vi "get_and_insert_SN.vi"(8 "error in (no error)":errorcluster, 10 "read buffer in":string, 11 "VISA Refnum in":refnum<visa-resource-name>) -> (0 "error out":errorcluster, 2 "read buffer out":string, 3 "VISA Refnum out":refnum<visa-resource-name>)   [LabVIEW 2015]
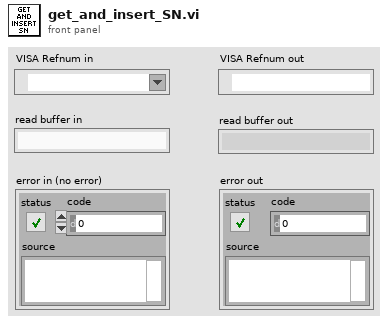
[diagram p1: front panel]
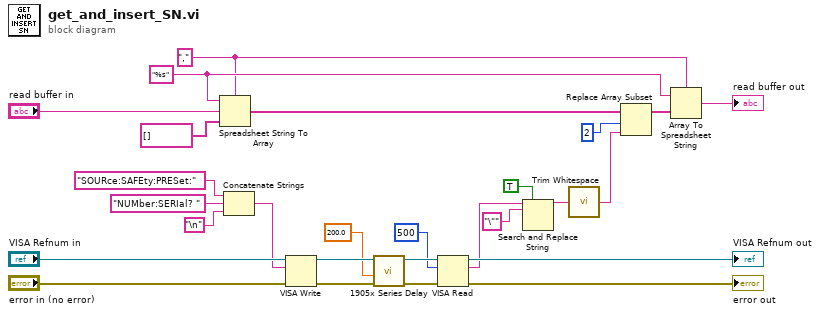
[diagram p0: block diagram]
diagram:
  w24 = "," ("delimiter (Tab)")
  w25 = "%s" ("format string")
  n1 = Spreadsheet String To Array(delimiter (Tab)=w24, format string=w25, spreadsheet string="read buffer in", array type (2D Dbl)=string[] []) -> (array=w14:string[])
  n2 = Concatenate Strings("SOURce:SAFEty:PRESet:", "NUMber:SERIal? ", "\n") -> (w5:string)
  n3 = VISA Write(VISA resource name="VISA Refnum in", write buffer=w5, error in (no error)="error in (no error)") -> (VISA resource name out=w26:refnum<visa-resource-name>, error out=w2:errorcluster)  [unwired: 1 out]
  n4 = call "1905x Series Delay.vi"("error in (no error)"=w2, "milliseconds to wait"=200.0) -> ("error out"=w3:errorcluster)  [unwired: 9 in]
  n5 = VISA Read(VISA resource name=w26, byte count=u32 500, error in (no error)=w3) -> (VISA resource name out=→"VISA Refnum out":refnum<visa-resource-name>, read buffer=w6:string, error out=→"error out":errorcluster)  [unwired: 1 out]
  n6 = Search and Replace String(replace all?=TRUE ("replace all? (F)"), input string=w6, search string="\"" ("substring (\"\")")) -> (result string=w16:string)  [unwired: 5 in, 3 out]
  n7 = call <vilib>:"Trim Whitespace.vi"("string"=w16) -> ("trimmed string"=w23:string)  [unwired: 1 in]
  n8 = Replace Array Subset(array=w14, new element=w23, index=2) -> (w21:string[])
  n9 = Array To Spreadsheet String(delimiter (Tab)=w24, array=w21, 3:w25) -> (spreadsheet string=→"read buffer out":string)
